vi "Get Master Data.vi"(8 "error in (no error)":errorcluster, 11 "EtherCAT Master in":T25 {"VS ref" format="%.0x"}) -> (0 "error out":errorcluster, 3 "ECAT Master out":T1 {"REM IO ECAT Slaves"."I/O Output Data"."BD Refs"."Data Reference" format="%.0x"; "REM IO ECAT Slaves"."I/O Input Data"."BD Refs"."Data Reference" format="%.0x"; "REM IO ECAT Slaves"."I/O Output Vars"."VS ref" format="%.0x"; "REM IO ECAT Slaves"."I/O Imput Vars"."VS ref" format="%.0x"; "REM IO ECAT Slaves"."VS ref" format="%.0x"; "Generic EtherCAT Slaves"."I/O Output Data"."BD Refs"."Data Reference" format="%.0x"; "Generic EtherCAT Slaves"."I/O Input Data"."BD Refs"."Data Reference" format="%.0x"; "Generic EtherCAT Slaves"."I/O Output Vars"."VS ref" format="%.0x"; "Generic EtherCAT Slaves"."I/O Imput Vars"."VS ref" format="%.0x"; "Generic EtherCAT Slaves"."VS ref" format="%.0x"; "VS ref" format="%.0x"; "EtherCAT Slaves"."FPGA"."VS ref" format="%.0x"; "EtherCAT Slaves"."RSI Modules"."VS ref" format="%.0x"; "EtherCAT Slaves"."VS ref" format="%.0x"})   [LabVIEW 2020, in "SEECD Engine.lvlib"]
uses:
  SEECD Engine.lvlib
  <vilib>/NI VeriStand/Custom Device API/Data Reference.ctl
  <vilib>/NI VeriStand/Custom Device API/Custom Device API.lvlib
  <vilib>/NI VeriStand/Custom Device API/Block Data Reference.ctl
  Type Defs/Output Data.ctl
  Type Defs/Input Data.ctl
  <vilib>/NI VeriStand/Custom Device API/Custom Device Item Ref.ctl
  Type Defs/FPGA Data.ctl
  Includes/Modules.lvlibp/RSI Module/RSI Module.lvclass
  Type Defs/RSI Module Data.ctl
  Type Defs/EtherCAT Slave Data.ctl
  Type Defs/EtherCAT Master Data.ctl
  Includes/Modules.lvlibp/RSI Module/Channel Type.ctl
  Shared/Type Defs/FXP Config.ctl
  Shared/SEECD Shared.lvlib
  Shared/Type Defs/UDV Data Type.ctl
  Type Defs/UDV Data.ctl
  Includes/Modules.lvlibp/RSI Module/Module Models.ctl
  Type Defs/Module Config Data.ctl
  Shared/Globals/Property Strings.vi
  Type Defs/Mixed IO.ctl
  Shared/Globals/RT Globals.vi
  Type Defs/Open Module IOVs.ctl
  Type Defs/Mod Size Indexes.ctl
  Type Defs/Generic ECAT Slave IOV Cluster.ctl
  Type Defs/Generic ECAT Slave Data Cluster.ctl
  Type Defs/Generic ECAT Slave RT-Data-Array.ctl
  <vilib>/NI VeriStand/Custom Device API/Get Item Property (U32).vi
  Type Defs/REM IO ECAT Slave IOV Cluster.ctl
  Type Defs/REM IO ECAT Slave Data Cluster.ctl
  Type Defs/REM IO ECAT Slave RT-Data-Array.ctl
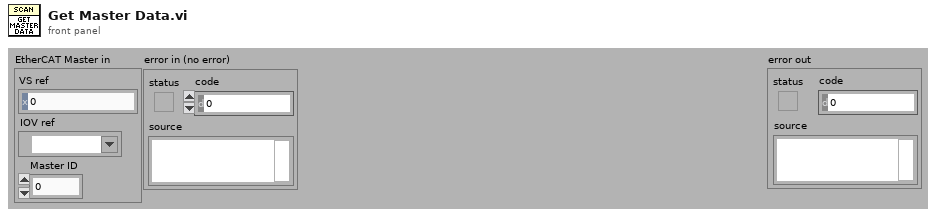
[diagram p1: front panel]
types:
  T1 = typedef "SEECD Engine.lvlib/EtherCAT Master Data.ctl" = cluster{"VS ref":T2, "IOV ref":refnum<k21>, "Master ID":u32, "Cyclic Data Bandwidth":u32, "EtherCAT Slaves":T3[], "Generic EtherCAT Slaves":T19, "REM IO ECAT Slaves":T22}
  T2 = typedef "Custom Device API.lvlib/Custom Device Item Ref.ctl" = u64
  T3 = typedef "SEECD Engine.lvlib/EtherCAT Slave Data.ctl" = cluster{"VS ref":T2, "IOV ref":refnum<k21>, "Position Address":u16, "RSI Modules":T4[], "FPGA":T14[], "Input Mod Size Idxs":T18, "Output Modules":i32[], "MixedIO Mod Size Idxs":T18}
  T4 = typedef "SEECD Engine.lvlib/RSI Module Data.ctl" = cluster{"VS ref":T2, "IOV ref":refnum<k21>, "Open Mod refs":T5, "Module DVR":refnum<data-value>, "Slot":u32, "Model":T6, "Channel Type":T7, "EtherCAT?":bool, "CDInput Data":T8, "CDOutput Data":T11, "Module Config Data":T12, "Mixed IO":T13}
  T5 = typedef "SEECD Engine.lvlib/Open Module IOVs.ctl" = cluster{"Analog Read":refnum<k21>, "Digital Read":refnum<k21>, "Analog Write":refnum<k21>, "Digital Write":refnum<k21>}
  T6 = typedef "Modules.lvlibp/RSI Module.lvclass/Module Models.ctl" = enum16{"Empty", "NI 9201", "NI 9203", "NI 9205", "NI 9206", "NI 9207", "NI 9208", "NI 9209", "NI 9210", "NI 9211", "NI 9212", "NI 9213", "NI 9214", "NI 9215", "NI 9216", "NI 9217", "NI 9219", "NI 9220", "NI 9221", "NI 9222", "NI 9223", "NI 9224", "NI 9225", "NI 9226", "NI 9227", "NI 9228", "NI 9229", "NI 9233", "NI 9234", "NI 9235", "NI 9236", "NI 9237", "NI 9239", "NI 9242", "NI 9244", "NI 9253", "NI 9263", "NI 9264", "NI 9265", "NI 9266", "NI 9269", "NI 9344", "NI 9350", "NI 9375", "NI 9401", "NI 9402", "NI 9403", "NI 9411", "NI 9421", "NI 9422", "NI 9423", "NI 9425", "NI 9426", "NI 9435", "NI 9436", "NI 9437", "NI 9472", "NI 9474", "NI 9475", "NI 9476", "NI 9477", "NI 9478", "NI 9481", "NI 9482", "NI 9485"}
  T7 = typedef "Modules.lvlibp/RSI Module.lvclass/Channel Type.ctl" = enum16{"Analog", "Digital"}
  T8 = typedef "SEECD Engine.lvlib/Input Data.ctl" = cluster{"BD Refs":T9[], "Data":dbl[], "Length":i32, "FIFO Index":i32}
  T9 = typedef "Custom Device API.lvlib/Block Data Reference.ctl" = cluster{"Data Reference":T10, "Offset":u64, "Length":u64}
  T10 = typedef "Custom Device API.lvlib/Data Reference.ctl" = i32
  T11 = typedef "SEECD Engine.lvlib/Output Data.ctl" = cluster{"BD Refs":T9[], "Length":i32, "FIFO Index":i32, "Data":dbl[]}
  T12 = typedef "SEECD Engine.lvlib/Module Config Data.ctl" = cluster{"Configurable?":bool, "Config Block Data Refs":T9[], "Config Data DVR":refnum<data-value>, "Previous Values":dbl[], "Local Reconfig VI Ref":refnum<vi>}
  T13 = typedef "SEECD Engine.lvlib/Mixed IO.ctl" = cluster{"Input Channel Indices":i32[], "Input Buffer":dbl[]}
  T14 = typedef "SEECD Engine.lvlib/FPGA Data.ctl" = cluster{"VS ref":T2, "IOV ref":refnum<k21>, "FPGA Target":enum16{"Local", "EtherCAT"}, "Product Code":u32, "Bitfile Signature":string, "Bitfile Path (RT)":path, "FPGA Session":u32, "Input Data":T8, "Output Data":T11, "UDVs":cluster{"From FPGA":T15[], "To FPGA":T15[]}}
  T15 = typedef "SEECD Engine.lvlib/UDV Data.ctl" = cluster{"VS ref":T2, "IOV Ref":refnum<k21>, "Name":string, "UDV Data Type":T16, "Supported Type?":bool, "FXP Config":T17, "FXP VI Ref":refnum<vi>}
  T16 = typedef "SEECD Shared.lvlib/UDV Data Type.ctl" = enum16{"Boolean", "Fixed Point", "Int8", "Int16", "Int32", "Int64", "U32 Bit Field", "UInt8", "UInt16", "UInt32", "UInt64", "Other", "DBL", "SGL"}
  T17 = typedef "SEECD Shared.lvlib/FXP Config.ctl" = cluster{"signed":bool, "size":u32, "integersize":i32}
  T18 = typedef "SEECD Engine.lvlib/Mod Size Indexes.ctl" = cluster{"4":i32[], "8":i32[], "16":i32[], "32":i32[], "other":i32[]}
  T19 = typedef "SEECD Engine.lvlib/Generic ECAT Slave RT-Data-Array.ctl" = T20[]
  T20 = typedef "SEECD Engine.lvlib/Generic ECAT Slave Data Cluster.ctl" = cluster{"VS ref":T2, "IOV ref":refnum<k21>, "Position Address":u16, "I/O Imput Vars ":T21[], "I/O Output Vars":T21[], "I/O Input Data":T8, "I/O Output Data":T11, "Distributed Clock":bool}
  T21 = typedef "SEECD Engine.lvlib/Generic ECAT Slave IOV Cluster.ctl" = cluster{"VS ref":T2, "IOV Ref":refnum<k21>, "Name":string, "UDV Data Type":T16}
  T22 = typedef "SEECD Engine.lvlib/REM IO ECAT Slave RT-Data-Array.ctl" = T23[]
  T23 = typedef "SEECD Engine.lvlib/REM IO ECAT Slave Data Cluster.ctl" = cluster{"VS ref":T2, "IOV ref":refnum<k21>, "Position Address":u16, "I/O Imput Vars ":T24[], "I/O Output Vars":T24[], "I/O Input Data":T8, "I/O Output Data":T11}
  T24 = typedef "SEECD Engine.lvlib/REM IO ECAT Slave IOV Cluster.ctl" = cluster{"VS ref":T2, "IOV Ref":refnum<k21>, "Name":string, "UDV Data Type":T16, "Scaling Factor":dbl}
  T25 = cluster{"VS ref":T2, "IOV ref":refnum<k21>, "Master ID":u32}
  T26 = cluster{"VS ref":T2, "IOV ref":refnum<k21>, "Position Address":u16}[]
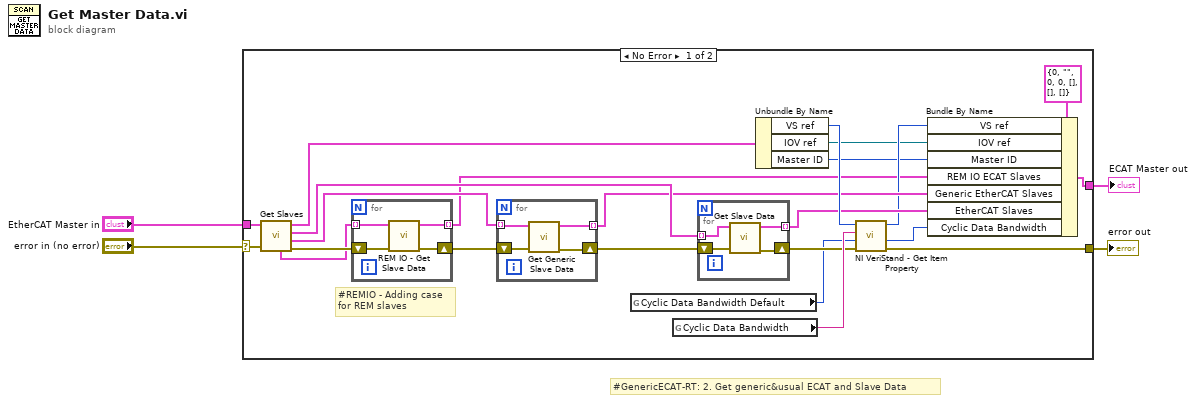
[diagram p0: block diagram]
diagram:
  # "#GenericECAT-RT: 2. Get generic&usual ECAT and Slave Data"
  n1 = case shown="No Error" "error in (no error)" {
    selector: "error in (no error)" -> [w13 w40]
    tunnel: "EtherCAT Master in" -> [w25 _]
    tunnel: [w24 _] -> w3
    tunnel: [w20 w40] -> w2
    frame No Error {
      # "#REMIO - Adding case for REM slaves"
      n2 = call "Get Slaves.vi"("error in (no error)"=w13, "EtherCAT Master in"=w25) -> ("error out"=w12:errorcluster, "ECAT Generic Slaves"=w18:T26, "ECAT Slaves"=w14:T26, "EtherCAT Master out"=w27:T25, "ECAT REM Slaves"=w10:T26)  [unwired: 5 in]
      n3 = for {
        shift-right: [w31] -> w11
        shift-left: w12 -> [w30]
        tunnel: w10 -> [w29] mode=indexing
        tunnel: [w28] -> w5 mode=indexing
        n4 = call "REM IO - Get Slave Data.vi"("error in (no error)"=w30, "EtherCAT Slave In"=w29) -> ("error out"=w31:errorcluster, "REM IO EtherCAT Slave"=w28:T23)  [unwired: 8 in]
      }
      n5 = for {
        shift-right: [w32] -> w17
        shift-left: w11 -> [w35]
        tunnel: w18 -> [w34] mode=indexing
        tunnel: [w33] -> w9 mode=indexing
        n6 = call "Get Generic Slave Data.vi"("error in (no error)"=w35, "EtherCAT Slave In"=w34) -> ("error out"=w32:errorcluster, "EtherCAT Slave out"=w33:T20)  [unwired: 8 in]
      }
      n7 = global read "RT Globals.vi" "Cyclic Data Bandwidth Default"() -> (w19:u32)
      n8 = global read "Property Strings.vi" "Cyclic Data Bandwidth"() -> (w23:string)
      n9 = for {
        tunnel: w14 -> [w38] mode=indexing
        shift-right: [w37] -> w22
        shift-left: w17 -> [w39]
        tunnel: [w36] -> w15 mode=indexing
        n10 = call "Get Slave Data.vi"("error in (no error)"=w39, "EtherCAT Slave in"=w38) -> ("error out"=w37:errorcluster, "EtherCAT Slave out"=w36:T3)  [unwired: 8 in]
      }
      n11 = Unbundle By Name(w27) -> ("VS ref"=w21:T2, "IOV ref"=w7:refnum<k21>, "Master ID"=w6:u32)
      n12 = call-poly <vilib>:"NI VeriStand - Get Item Property.vi"("error in (no error)"=w22, "Default Value"=w19, "Property Name"=w23, "Item Ref in"=w21) -> ("error out"=w20:errorcluster, "Value"=w16:u32, "Item Ref out"=w8:T2)  [unwired: 4 in, 1 out]
      n13 = Bundle By Name(cluster=T1 {"VS ref"=0, "IOV ref"="", "Master ID"=0, "Cyclic Data Bandwidth"=0, "EtherCAT Slaves"=[], "Generic EtherCAT Slaves"=[], "REM IO ECAT Slaves"=[]} ("EtherCAT Master"), "VS ref"=w8, "IOV ref"=w7, "Master ID"=w6, "REM IO ECAT Slaves"=w5, "Generic EtherCAT Slaves"=w9, "EtherCAT Slaves"=w15, "Cyclic Data Bandwidth"=w16) -> (w24:T1)
    }
    frame Error {
    }
  }
  "ECAT Master out" <- w3
  "error out" <- w2
